vi "Write Meta.vi"(8 "error in":errorcluster, 10 "Variables":cluster{"name":string, "type desc":i16[]}[](array[cluster]), 11 "connection ID":refnum<k5>) -> (0 "error out":errorcluster, 3 "connection ID out":refnum<k5>)   [LabVIEW 2010]
doc: "Use this VI to transmit the Meta data cluster to a remote computer via TCP/IP. Sending the meta data to another computers helps maintainability since the data resides only on one side and itis shared to other computers at run time.\n\nThe meta data cluster must contain valid name and type information before being sent.\n\nThis VI converts the meta data cluster into XML format before transfering it to a remote computer. If your application communicates with a non-LabVIEW program, you can still use this VI but make sure the receiving code knows how to parse through the XML string."
panel:
  out "XML Source Text (Simple Food Menu found on Web)":string="<?xml version=\"1.0\" encoding=\"ISO8859-1\" ?>\n<breakfast-menu>\n  <food>\n    <name>Belgian Waffles</name>\n    <price>$5.95</price>\n    <description>two of our famous Belgian Waffles with plenty of real maple syrup</description>\n    <calories>650</calories>\n  </food>\n  <food>\n    <name>Strawberry Belgian Waffles</name>\n    <price>$7.95</price>\n    <description>light Belgian waffles covered with strawberrys and whipped cream</description>\n    <calories>900</calories>\n  </food>\n  <food>\n    <name>Berry-Berry Belgian Waffles</name>\n    <price>$8.95</price>\n    <description>light Belgian waffles covered with an assortment of fresh berries and whipped cream</description>\n    <calories>900</calories>\n  </food>\n  <food>\n    <name>French Toast</name>\n    <price>$4.50</price>\n    <description>thick slices made from our homemade sourdough bread</description>\n    <calories>600</calories>\n  </food>\n  <food>\n    <name>Homestyle Breakfast</name>\n    <price>$6.95</price>\n    <description>two eggs, bacon or sausage, toast, and our ever-popular hash browns</description>\n    <calories>950</calories>\n  </food>\n</breakfast-menu>"
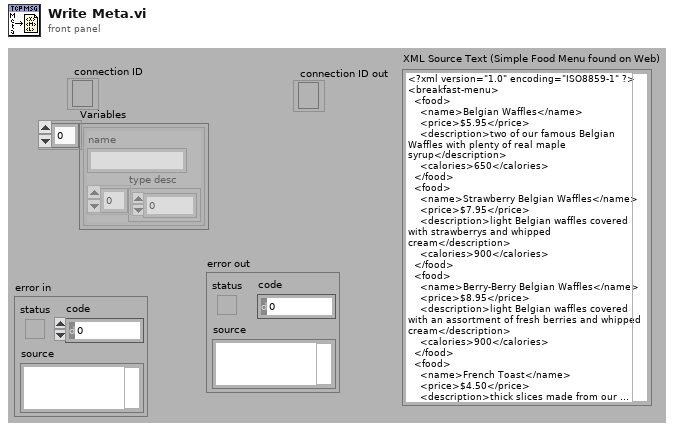
[diagram p1: front panel]
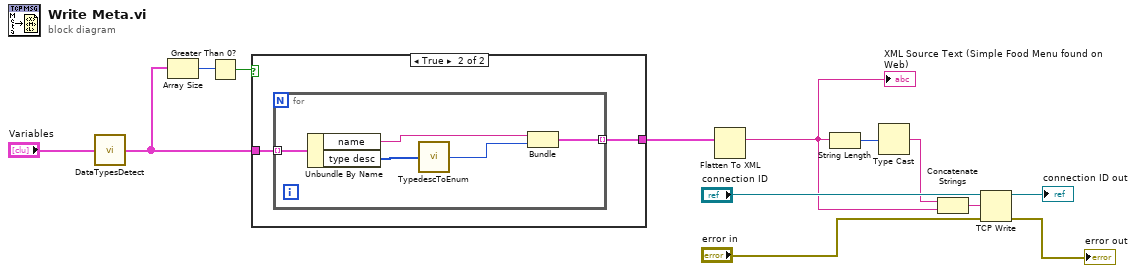
[diagram p0: block diagram]
diagram:
  n1 = call "DataTypesDetect.vi"("input data"="Variables") -> ("output data"=w1:cluster{"name":string, "type desc":i16[]}[])
  n2 = Array Size(array=w1) -> (size(s)=w5:i32)
  n3 = Greater Than 0?(x=w5) -> (x > 0?=w4:bool)
  n4 = case shown="True" w4 {
    tunnel: w1 -> [_ w15]
    tunnel: [_ w14] -> w3
    frame False {
    }
    frame True {
      n5 = for {
        tunnel: w15 -> [w20] mode=indexing
        tunnel: [w16] -> w14 mode=indexing
        n6 = Unbundle By Name(w20) -> ("name"=w18:string, "type desc"=w19:i16[])
        n7 = call "TypedescToEnum.vi"("type desc"=w19) -> ("DataType"=w17:u16)
        n8 = Bundle("name"=w18, "DataType"=w17) -> (w16:cluster{"name":string, "DataType":u16})  [unwired: 1 out]
      }
    }
  }
  n9 = Flatten To XML(anything=w3) -> (xml string=w6:string)
  "XML Source Text (Simple Food Menu found on Web)" <- w6
  n10 = String Length(string=w6) -> (length=w9:i32)
  n11 = Type Cast(x=w9) -> (*(type *) &x=w10:string)  [unwired: 1 out]
  n12 = Concatenate Strings(w10, w6) -> (w11:string)
  n13 = TCP Write(connection ID="connection ID", data in=w11, error in (no error)="error in") -> (connection ID out=→"connection ID out":refnum<k5>, error out=→"error out":errorcluster)  [unwired: 2 out]
